vi "WSVCAP SHL Host TL I2C Configure.vi"(0 "I2C_Slave Address":u8=20, 9 "Clock Rate (Hz)":dbl=50000.0, 11 "error in":errorcluster, 13 "Log (T)":bool=TRUE) -> (6 "Actual Rate (Hz)":dbl, 15 "error out":errorcluster)   [LabVIEW 2012]
uses:
  Type Defs/WSVCAP SHL Function Enum.ctl
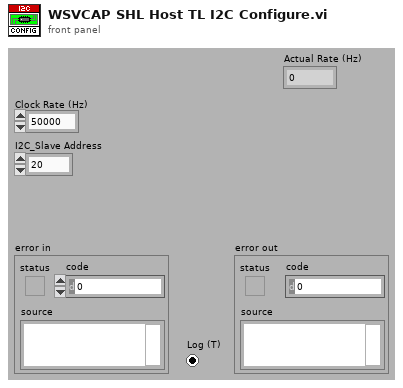
[diagram p1: front panel]
types:
  T1 = typedef "WSVCAP SHL Function Enum.ctl" = enum16{"Initialize", "Configure I2C", "Configure SPI", "Configure RFFE", "Write I2C", "Read I2C", "Write/Read SPI", "Start SPI Cycle", "Stop SPI Cycle", "Write RFFE", "Read RFFE", "Start RFFE Cycle", "Stop RFFE Cycle", "Get Status", "Close"}
  T2 = typedef "WSVCAP SHL Core System Cluster.ctl" = cluster{"Settings":T3, "FPGA Resource":tag, "Online":bool, "I2C Wait Ticks":u32, "SPI Wait Ticks":u32, "RFFE Wait Ticks":u32}
  T3 = typedef "WSVCAP SHL I2C Settings Cluster.ctl" = cluster{"FPGA Resource Name":string, "I2C Slave Address":u8, "I2C Clock Rate (Hz)":dbl, "SPI Clock Rate (Hz)":dbl, "RFFE Slave Address":u8, "RFFE Clock Rate (Hz)":dbl, "Simulate FPGA":bool}
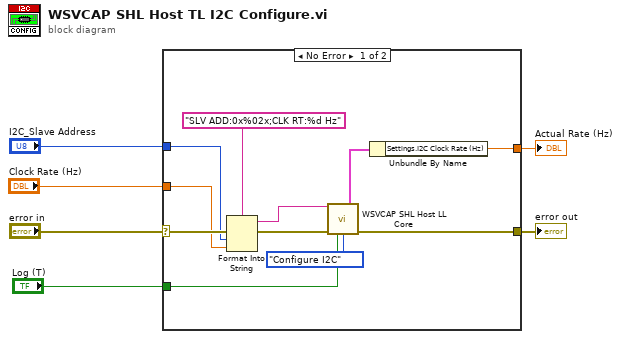
[diagram p0: block diagram]
diagram:
  n1 = case shown="No Error" "error in" {
    selector: "error in" -> [w15 w18]
    tunnel: [w17 w18] -> w5
    tunnel: "Clock Rate (Hz)" -> [w13 _]
    tunnel: "I2C_Slave Address" -> [w12 _]
    tunnel: [w9 _] -> w2
    tunnel: "Log (T)" -> [w7 _]
    frame No Error {
      n2 = Format Into String(format string="SLV ADD:0x%02x;CLK RT:%d Hz", error in=w15, w12, w13) -> (resulting string=w11:string, error out=w14:errorcluster)  [unwired: 1 in]
      n3 = call "WSVCAP SHL Host LL Core.vi"("Message In"=w11, "error in"=w14, "Log (T)"=w7, "Function"=WSVCAP_SHL_Function_Enum."Configure I2C") -> ("System"=w10:T2, "error out"=w17:errorcluster)  [unwired: 9 in, 1 out]
      n4 = Unbundle By Name(w10) -> ("Settings.I2C Clock Rate (Hz)"=w9:dbl)
    }
    frame Error {
    }
  }
  "Actual Rate (Hz)" <- w2
  "error out" <- w5
